vi "Write Cell string and Format Border.vi"(8 "error in (no error)":errorcluster, 9 "output cluster":cluster{"row":i32, "column":i32}, 10 "input string":string, 11 "NI_report in":refnum<class "NI_report.lvclass">) -> (0 "error out":errorcluster, 3 "NI_report out":refnum<class "NI_report.lvclass">)   [LabVIEW 2016]
uses:
  <vilib>/Utility/NIReport.llb/NI_report.lvclass
  <vilib>/addons/_office/NI_ReportGenerationToolkit.lvlib
  <vilib>/Utility/NIReport.llb/Excel/NI_Excel.lvclass
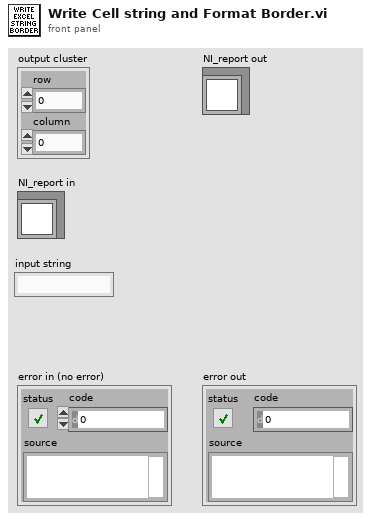
[diagram p1: front panel]
types:
  T1 = cluster{"on/off":bool, "weight":i32, "color":u32}
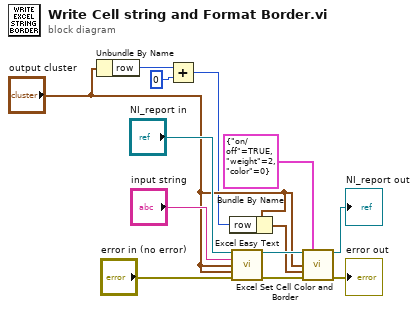
[diagram p0: block diagram]
diagram:
  n1 = Unbundle By Name("output cluster") -> ("row"=w3:i32)
  n2 = Add(x=w3, y=0) -> (x+y=w2:i32)
  n3 = Bundle By Name(cluster="output cluster", "row"=w2) -> (w4:cluster{"row":i32, "column":i32})
  n4 = call <vilib>:"Excel Easy Text.vi"("report in"="NI_report in", "text"="input string", "start (-1, -1)"="output cluster", "end (-1, -1)"="output cluster", "error in (no error)"="error in (no error)") -> ("report out"=w12:refnum<class "NI_report.lvclass">, "error out"=w10:errorcluster)  [unwired: 6 in, 3 out]
  n5 = call <vilib>:"Excel Set Cell Color and Border.vi"("report in"=w12, "inside border"=T1 {"on/off"=TRUE, "weight"=2, "color"=0}, "start (-1, -1)"="output cluster", "end (-1, -1)"=w4, "error in (no error)"=w10) -> ("report out"=→"NI_report out":refnum<class "NI_report.lvclass">, "error out"=→"error out":errorcluster)  [unwired: 9 in]
